vi "Deadzone.vi"(8 "error in (no error)":errorcluster, 10 "Deadzone":dbl, 11 "Input":dbl) -> (0 "error out":errorcluster, 1 "Just entered deadzone?":bool, 2 "In deadzone?":bool, 3 "Output":dbl)   [LabVIEW 2015]
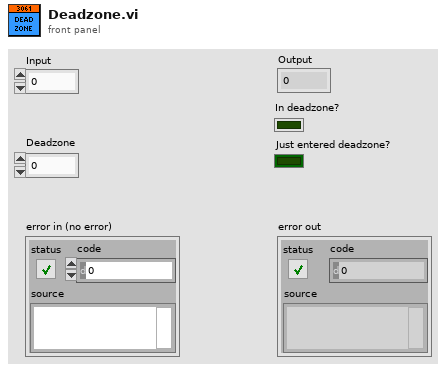
[diagram p1: front panel]
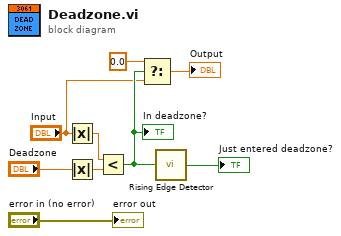
[diagram p0: block diagram]
diagram:
  n1 = Absolute Value(x="Input") -> (abs(x)=w8:dbl)
  n2 = Absolute Value(x="Deadzone") -> (abs(x)=w6:dbl)
  n3 = Less?(x=w8, y=w6) -> (x < y?=w4:bool)
  "In deadzone?" <- w4
  n4 = Select(t=0.0, s=w4, f="Input") -> (s? t:f=→"Output":dbl)
  n5 = call "Rising Edge Detector.vi"("Input"=w4) -> ("Rising edge?"=→"Just entered deadzone?":bool)
  "error out" <- "error in (no error)"
